vi "Execute.vi"(6 "Index [-1]":i32=-1, 7 "Composite Object":refnum<class "CConfig Object.lvclass">, 8 "error in (no error)":errorcluster, 9 "Results":string[][](array[string]), 11 "Config Query in":refnum<class "Step In Query.lvclass">) -> (0 "error out":errorcluster, 1 "Results":string[][](array[string]), 2 "Result":bool, 3 "Config Query out":refnum<class "Step In Query.lvclass">, 4 "Index":i32, 5 "Composite Object":refnum<class "CConfig Object.lvclass">)   [LabVIEW 2013, in "Step In Query.lvclass"]
doc: "Copyright 2018, Carya Automatisering, Wiebe Walstra."
uses:
  Step In Query.lvclass
  CConfig Object.lvclass
  Step In Query.lvclass/Step In Query.ctl
  CConfig Query.lvclass
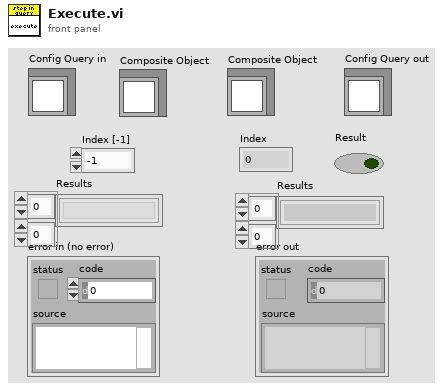
[diagram p1: front panel]
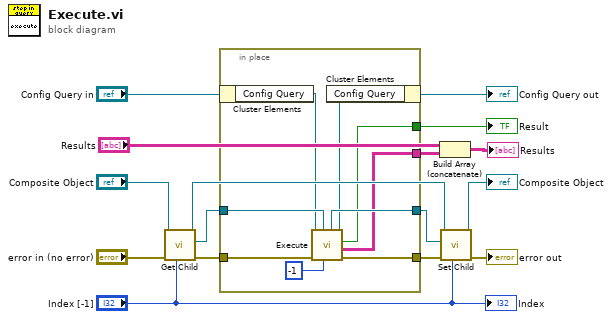
[diagram p0: block diagram]
diagram:
  n1 = call-dynamic "Get Child.vi"("Index in"="Index [-1]", "error in (no error)"="error in (no error)", "Composite Object in"="Composite Object") -> ("error out"=w15:errorcluster, "Child"=w10:refnum<class "CConfig Object.lvclass">, "Composite Object out"=w8:refnum<class "CConfig Object.lvclass">)  [unwired: 6 in]
  n2 = in-place {
    in-place-border: w15 -> [w25]
    in-place-border: [w24] -> w11
    in-place-border: w10 -> [w23]
    in-place-border: [w22] -> w9
    in-place-border: [w21] -> w7
    in-place-border: [w18] -> w4
    n3 = in-place-cluster #1("Config Query in") -> ("Config Query"=w20:refnum<class "CConfig Query.lvclass">)
    n4 = call-dynamic "Execute.vi"("Index [-1]"=-1, "Composite Object"=w23, "error in (no error)"=w25, "Config Query in"=w20) -> ("error out"=w24:errorcluster, "Results"=w18:string[][], "Result"=w21:bool, "Config Query out"=w19:refnum<class "CConfig Query.lvclass">, "Composite Object"=w22:refnum<class "CConfig Object.lvclass">)  [unwired: 2 in, 1 out]
    n5 = in-place-cluster #1("Config Query"=w19) -> (→"Config Query out":refnum<class "Step In Query.lvclass">)
  }
  "Result" <- w7
  n6 = Build Array (concatenate)("Results", w4) -> (→"Results":string[][])
  n7 = call-dynamic "Set Child.vi"("Index in"="Index [-1]", "error in (no error)"=w11, "Child"=w9, "Composite Object in"=w8) -> ("error out"=→"error out":errorcluster, "Composite Object out"=→"Composite Object":refnum<class "CConfig Object.lvclass">)  [unwired: 6 in]
  "Index" <- "Index [-1]"
